vi "Highlight Execution.vi"(8 "error in (no error)":errorcluster, 9 "Highlight Execution?":bool, 10 "VIs":string[](array[string]), 11 "Application in":refnum<vi>) -> (0 "error out":errorcluster)   [LabVIEW 2013, in "LVTM.lvlib"]
uses:
  LVTM.lvlib
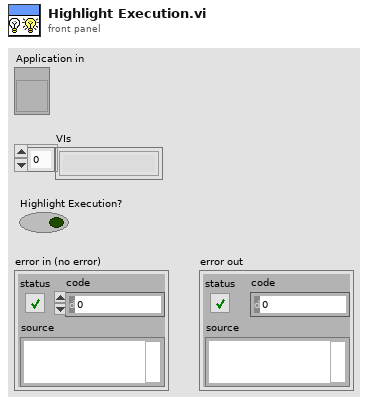
[diagram p1: front panel]
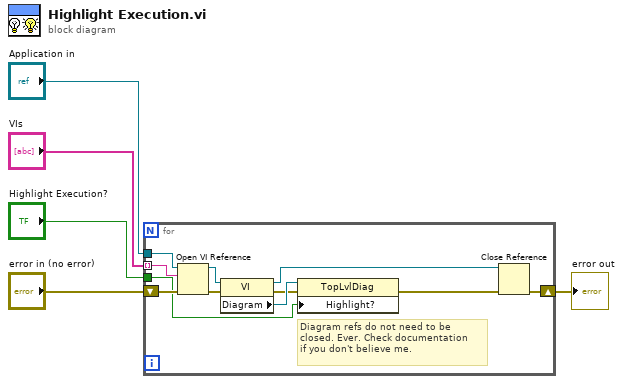
[diagram p0: block diagram]
diagram:
  n1 = for {
    tunnel: "VIs" -> [w14] mode=indexing
    shift-right: [w16] -> w2
    shift-left: "error in (no error)" -> [w15]
    tunnel: "Application in" -> [w7]
    tunnel: "Highlight Execution?" -> [w6]
    # "Diagram refs do not need to be\nclosed. Ever. Check documentation\nif you don't believe me."
    n2 = Open VI Reference(application reference (local)=w7, vi path=w14, error in (no error)=w15) -> (vi reference=w12:refnum<vi>, error out=w13:errorcluster)  [unwired: 3 out]
    n3 = property class="VI"(reference=w12, error in=w13) -> (reference out=w11:refnum<vi>, error out=w9:errorcluster, "Diagram"=w10:refnum<vi>)
    n4 = property class="TopLvlDiag"(reference=w10, error in=w9, "Highlight?"=w6) -> (error out=w8:errorcluster)  [unwired: 1 out]
    n5 = Close Reference(reference=w11, error in (no error)=w8) -> (error out=w16:errorcluster)
  }
  "error out" <- w2
